vi "Spring Motor Main.vi"() -> ()   [LabVIEW 2021]
uses:
  Spring Motor.lvclass
  Communication/Comm/Comm.lvclass
  Communication/Serial/Serial.lvclass
  Communication/Wifi/Wifi.lvclass
panel:
  in  "Horizontal Pointer Slide":u32(slide) scale=0.0..180.0
  out "Error Status":errorcluster
  out "Command Sucessful?":bool
  out "Echo":string
  in  "Angle (Deg)":dbl
  in  "Turn Motor on":bool
  in  "Stop":bool
  out "Motor Signal":dbl(graph)
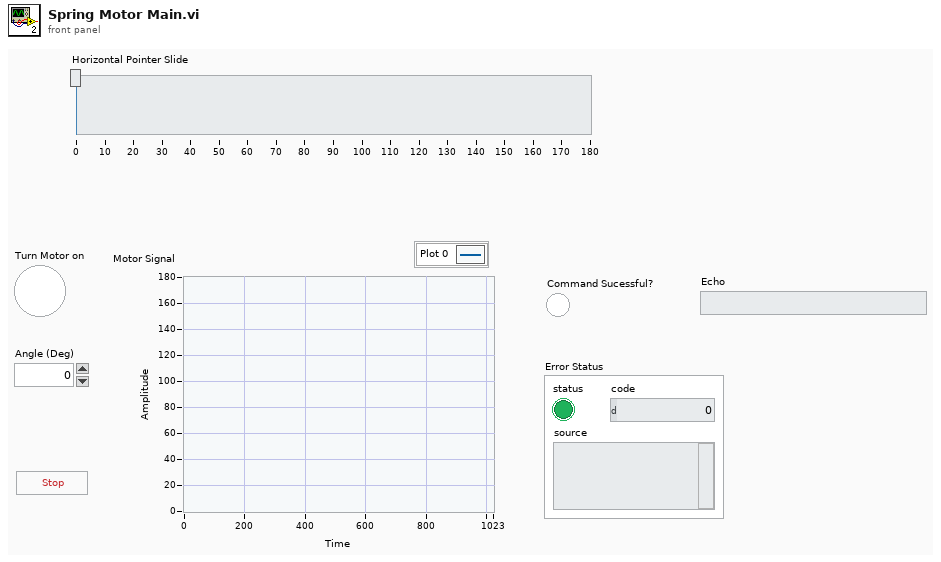
[diagram p1: front panel]
types:
  T1 = enum8{"Enabled", "Disabled", "Disabled and Grayed Out"}
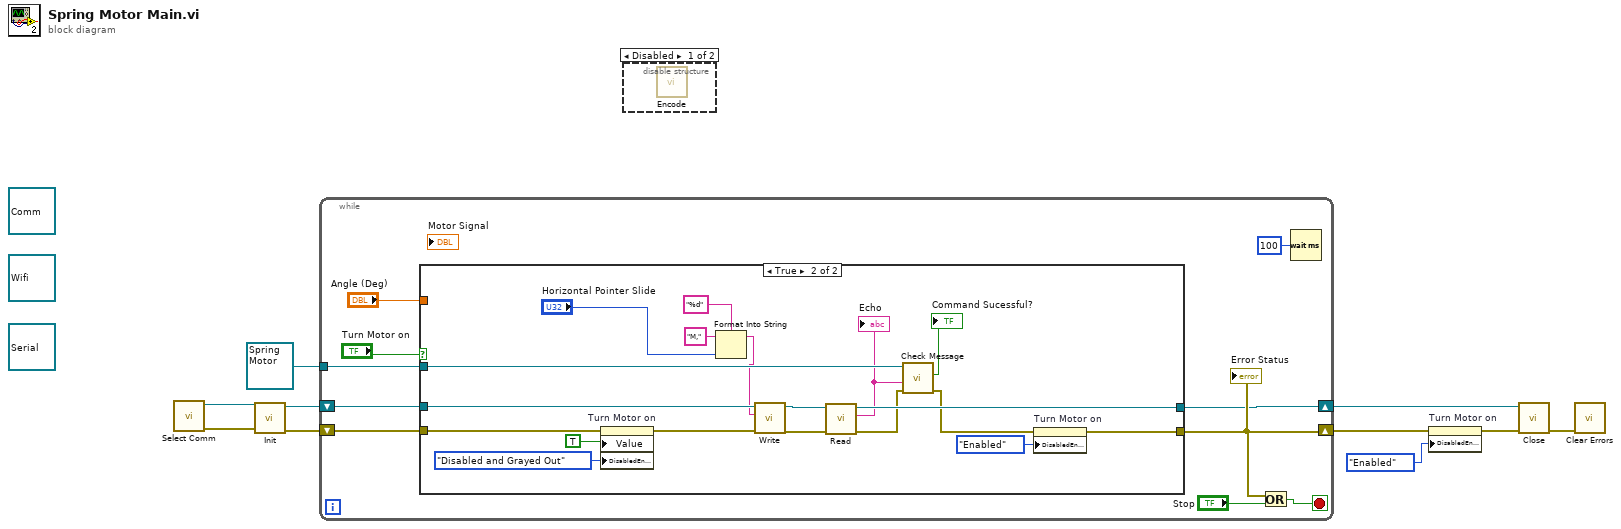
[diagram p0: block diagram]
diagram:
  (unwired) refnum<class "Wifi.lvclass"> refnum ("Wifi.lvclass")
  (unwired) refnum<class "Serial.lvclass"> refnum ("Serial.lvclass")
  (unwired) refnum<class "Comm.lvclass"> refnum ("Comm in")
  n1 = call "Select Comm.vi"() -> ("error out"=w7:errorcluster, "Comm.lvclass"=w8:refnum<class "Comm.lvclass">)  [unwired: 10 in]
  n2 = call-dynamic "Init.vi"("error in (no error)"=w7, "Comm in"=w8) -> ("error out"=w10:errorcluster, "Comm out"=w9:refnum<class "Comm.lvclass">)  [unwired: 8 in]
  n3 = while {
    shift-right: [w15] -> w2
    shift-left: w10 -> [w12]
    shift-right: [w14] -> w1
    shift-left: w9 -> [w13]
    tunnel: refnum<class "Spring Motor.lvclass"> refnum ("Spring Motor in") -> [w18]
    stop <- w16 stop-if-true
    n4 = case shown="True" "Turn Motor on" {
      tunnel: w18 -> [_ w41]
      tunnel: [w21 w28] -> w15
      tunnel: [w22 w37] -> w14
      tunnel: w13 -> [w22 w36]
      tunnel: w12 -> [w21 w33]
      tunnel: "Angle (Deg)" -> [_ _]
      frame False {
      }
      frame True {
        n5 = property on="Turn Motor on" class="Bool (strict)"(error in=w33, "Value"=TRUE ("Turn Motor on"), "DisabledEnum"=T1."Disabled and Grayed Out" ("Disabled")) -> (error out=w34:errorcluster)  [unwired: 1 in, 1 out]
        n6 = Format Into String(format string="%d", initial string="M,", "Horizontal Pointer Slide") -> (resulting string=w23:string)  [unwired: 1 in, 1 out]
        n7 = call-dynamic "Write.vi"("error in (no error)"=w34, "Message"=w23, "Comm in"=w36) -> ("error out"=w39:errorcluster, "Comm out"=w38:refnum<class "Comm.lvclass">)  [unwired: 7 in]
        n8 = call-dynamic "Read.vi"("error in (no error)"=w39, "Comm in"=w38) -> ("error out"=w31:errorcluster, "Message"=w32:string, "Comm out"=w37:refnum<class "Comm.lvclass">)  [unwired: 7 in]
        "Echo" <- w32
        n9 = call-dynamic "Check Message.vi"("error in (no error)"=w31, "Echo Received"=w32, "Actuator in"=w41) -> ("error out"=w30:errorcluster, "Command Sucessful?"=→"Command Sucessful?":bool)  [unwired: 6 in, 1 out]
        n10 = property on="Turn Motor on" class="Bool (strict)"(error in=w30, "DisabledEnum"=T1."Enabled" ("Disabled")) -> (error out=w28:errorcluster)  [unwired: 1 in, 1 out]
      }
    }
    "Error Status" <- w15
    n11 = Or(x=w15, y="Stop") -> (x .or. y?=w16:bool)
    n12 = Wait (ms)(milliseconds to wait=u32 100) -> ()  [unwired: 1 out]
  }
  n13 = disable-structure shown="Disabled" {
    frame Disabled {
      n14 = call-dynamic "Encode.vi"() -> ()  [unwired: 9 in, 3 out]
    }
    frame Enabled {
    }
  }
  n15 = property on="Turn Motor on" class="Bool (strict)"(error in=w2, "DisabledEnum"=T1."Enabled" ("Disabled")) -> (error out=w3:errorcluster)  [unwired: 1 in, 1 out]
  n16 = call-dynamic "Close.vi"("error in (no error)"=w3, "Comm in"=w1) -> ("error out"=w5:errorcluster)  [unwired: 8 in, 1 out]
  n17 = call <vilib>:"Clear Errors.vi"("error in (no error)"=w5) -> ()  [unwired: 5 in, 2 out]
